vi "Write ClassID.vi"(5 "ClassID":u32, 9 "Generic in":refnum<class "Generic.lvclass">) -> (3 "Generic out":refnum<class "Generic.lvclass">)   [LabVIEW 2014, in "Raspberry Pi Compatible Compiler for LabVIEW.lvlib" / "Generic.lvclass"]
uses:
  Generic.lvclass
  Generic.lvclass/Generic.ctl
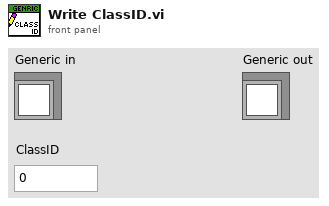
[diagram p1: front panel]
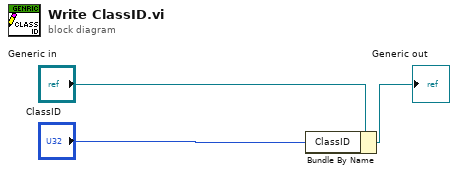
[diagram p0: block diagram]
diagram:
  n1 = Bundle By Name(cluster="Generic in", "ClassID"="ClassID") -> (→"Generic out":refnum<class "Generic.lvclass">)
